vi "InitServo.vi"(3 "error in":errorcluster) -> (0 "error out":errorcluster, 1 "Device Connection Cluster":T1, 2 "Boolean":bool)   [LabVIEW 2013]
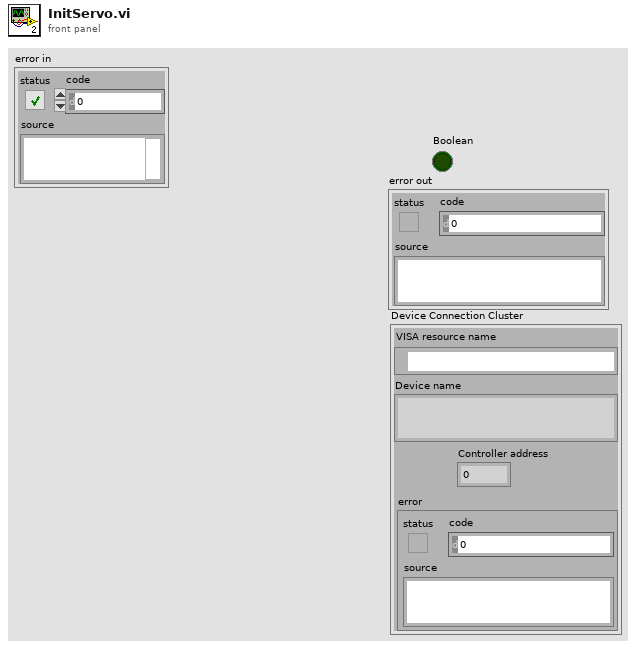
[diagram p1: front panel]
types:
  T1 = cluster{"VISA resource name":refnum<visa-resource-name>, "Device name":string, "Controller address":i32, "error":errorcluster}
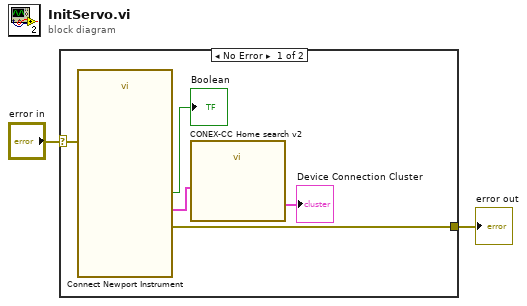
[diagram p0: block diagram]
diagram:
  n1 = case shown="No Error" "error in" {
    selector: "error in" -> [w6 w8]
    tunnel: [w5 w8] -> w1
    frame No Error {
      n2 = call <userlib>:"Connect Newport Instrument.vi"("error in (no error)"=w6) -> ("error (duplicate)"=w5:errorcluster, "Connected"=→"Boolean":bool, "Device Connection Cluster"=w4:T1)  [unwired: 6 in, 2 out]
      n3 = call <userlib>:"CONEX-CC Home search v2.vi"("Connection Cluster in"=w4) -> ("Connection Cluster out"=→"Device Connection Cluster":T1)  [unwired: 8 in]
    }
    frame Error {
    }
  }
  "error out" <- w1
